vi "Publish Client List.vi"(8 "error in (no error)":errorcluster, 11 "Messaging Server Module in":refnum<class "Messaging Server Module.lvclass">) -> (0 "error out":errorcluster, 3 "Messaging Server Module out":refnum<class "Messaging Server Module.lvclass">)   [LabVIEW 2020, in "Volatus.lvlib" / "Messaging Server Module.lvclass"]
uses:
  Messaging Server Module.lvclass
  Messaging Server Module.lvclass/Messaging Server Module.ctl
  Msg Client State.ctl
  Volatus.lvlib
  lv-vecto/Vecto/proto/TcpClientInfo/Data.ctl
  lv-vecto/Vecto/proto/TcpClientInfo/TcpClientInfo.lvlib
  lv-vecto/Vecto/proto/TcpClientList/Data.ctl
  lv-vecto/Vecto/proto/TcpClientList/TcpClientList.lvlib
  Module/Module.lvclass
  lv-vecto/Vecto/proto/TcpClientList/Class/Msg.lvclass
  C:/dev/lv20CE/relink/lv-volatus/Volatus/Module/Module.lvclass
  C:/dev/lv20CE/relink/lv-volatus/Volatus/Messaging Server Module/Messaging Server Module.lvclass
  VolatusAPI/VolatusAPI.lvclass
  C:/dev/lv20CE/relink/lv-vecto/Vecto/proto/TcpClientList/Class/Msg.lvclass
  C:/dev/lv20CE/relink/lv-protoc/LV-Proto/Message/Message.lvclass
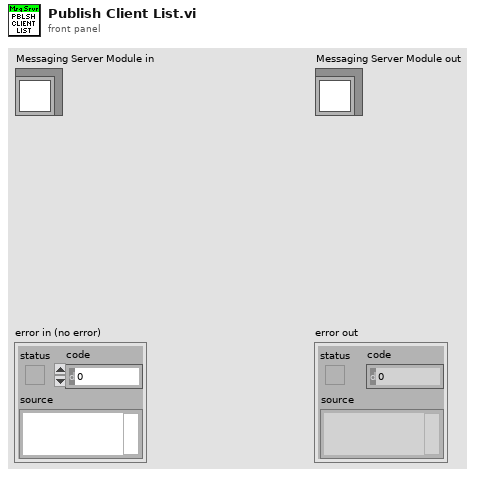
[diagram p1: front panel]
types:
  T1 = typedef "TcpClientList.lvlib/Data.ctl" = cluster{"clients":T2[]}
  T2 = typedef "TcpClientInfo.lvlib/Data.ctl" = cluster{"node_id":u32, "node_name":string, "app_version":string, "config_version":string, "config_hash":string, "node_alias":string, "address":string}
  T3 = typedef "Volatus.lvlib/Messaging Server Module.lvclass/Client Info.ctl" = cluster{"MsgQ":refnum<class "MessageQ.lvclass">, "Address":string, "Port":u16, "Client State":T4, "Last Update":dbl, "TCP":refnum<k5>, "Details":T2}
  T4 = typedef "Volatus.lvlib/Msg Client State.ctl" = enum16{"Unknown", "Handshake", "Connected", "Closing"}
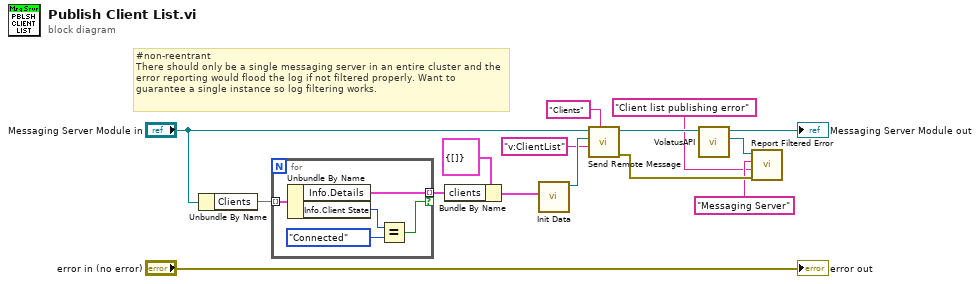
[diagram p0: block diagram]
diagram:
  # "#non-reentrant\nThere should only be a single messaging server in an entire cluster and the error reporting would flood the log if not filtered properly. Want to guarantee a single instance so log filtering works."
  n1 = Unbundle By Name("Messaging Server Module in") -> ("Clients"=w12:map{string, T3})
  n2 = for {
    tunnel: w12 -> [w20] mode=indexing
    tunnel: [w16] -> w10 mode=indexing if=w17
    n3 = Unbundle By Name(w20) -> ("Info.Details"=w16:T2, "Info.Client State"=w19:T4)
    n4 = Equal?(x=w19, y=Msg_Client_State."Connected") -> (x = y?=w17:bool)
  }
  n5 = Bundle By Name(cluster=T1 {"clients"=[]} ("Data"), "clients"=w10) -> (w7:T1)
  n6 = call "Init Data.vi"("Data"=w7) -> ("Msg out"=w6:refnum<class "Msg.lvclass">)  [unwired: 10 in]
  n7 = call "Send Remote Message.vi"("Target Name"="Clients", "Message Type"="v:ClientList", "Message"=w6, "Module in"="Messaging Server Module in") -> ("error out"=w15:errorcluster, "Module out"=w9:refnum<class "Messaging Server Module.lvclass">)  [unwired: 6 in]
  n8 = call "VolatusAPI.vi"("Module in"=w9) -> ("VolatusAPI"=w3:refnum<class "VolatusAPI.lvclass">, "Module out"=→"Messaging Server Module out":refnum<class "Messaging Server Module.lvclass">)  [unwired: 9 in]
  n9 = call "Report Filtered Error.vi"("error in (no error)"=w15, "Message"="Client list publishing error", "Context"="Messaging Server", "VolatusAPI in"=w3) -> ()  [unwired: 6 in, 2 out]
  "error out" <- "error in (no error)"
